vi "isUserOperator.vi"(11 "Sequence Context":T1) -> (2 "Operator":bool)   [LabVIEW 2025]
uses:
  <vilib>/addons/TestStand/_TSLegacy.llb/LabVIEW Test - Sequence Context.ctl
panel:
  out "error out":errorcluster
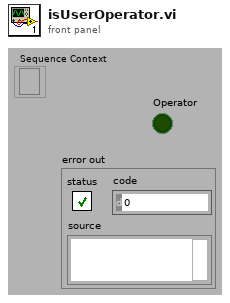
[diagram p1: front panel]
types:
  T1 = typedef "LabVIEW Test - Sequence Context.ctl" = refnum<k7>
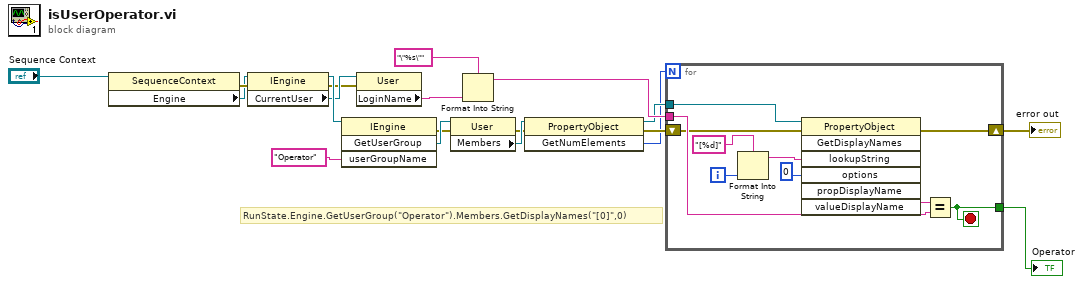
[diagram p0: block diagram]
diagram:
  # "RunState.Engine.GetUserGroup(\"Operator\").Members.GetDisplayNames(\"[0]\",0)"
  n1 = property class="SequenceContext"(reference="Sequence Context") -> (error out=w18:errorcluster, "Engine"=w17:refnum<k7>)  [unwired: 1 in, 1 out]
  n2 = property class="IEngine"(reference=w17, error in=w18) -> (reference out=w16:refnum<k7>, error out=w11:errorcluster, "CurrentUser"=w15:refnum<k7>)
  n3 = invoke class="IEngine" method="GetUserGroup"(reference=w16, "userGroupName"="Operator") -> (error out=w6:errorcluster, "GetUserGroup"=w9:refnum<k7>)  [unwired: 2 in, 2 out]
  n4 = property class="User"(reference=w15, error in=w11) -> ("LoginName"=w14:string)  [unwired: 2 out]
  n5 = property class="User"(reference=w9, error in=w6) -> (error out=w5:errorcluster, "Members"=w8:refnum<k7>)  [unwired: 1 out]
  n6 = Format Into String(format string="\"%s\"", w14) -> (resulting string=w12:string)  [unwired: 2 in, 1 out]
  n7 = invoke class="PropertyObject" method="GetNumElements"(reference=w8, error in=w5) -> (reference out=w7:refnum<k7>, error out=w4:errorcluster, "GetNumElements"=w3:i32)  [unwired: 1 in]
  n8 = for {
    N: w3 -> [_]
    tunnel: w7 -> [w29]
    tunnel: w12 -> [w24]
    tunnel: [w20] -> w1
    shift-right: [w21] -> w10
    shift-left: w4 -> [w22]
    i -> [w23]
    stop <- w20 stop-if-true
    n9 = Format Into String(format string="[%d]", w23) -> (resulting string=w27:string)  [unwired: 2 in, 1 out]
    n10 = invoke class="PropertyObject" method="GetDisplayNames"(reference=w29, error in=w22, "lookupString"=w27, "options"=0) -> (error out=w21:errorcluster, "valueDisplayName"=w25:string)  [unwired: 3 in, 5 out]
    n11 = Equal?(x=w25, y=w24) -> (x = y?=w20:bool)
  }
  "error out" <- w10
  "Operator" <- w1
